vi "ARCOS-- Check  Missing Dependent VI.vi"() -> ()   [LabVIEW 2020]
panel:
  out "DependentVI File":path
  out "ComparedVIs":cluster{string, bool}[](array[cluster])
  out "Missing VIs":string[](array[string])
  out "ExternalAddOn":string[](array[string])
  in  "vi path Compare":path=path "D:/Project/ARCOS2020/ExternalModules/USERCallVISample.vi"
  in  "ARCOSMainVI":path
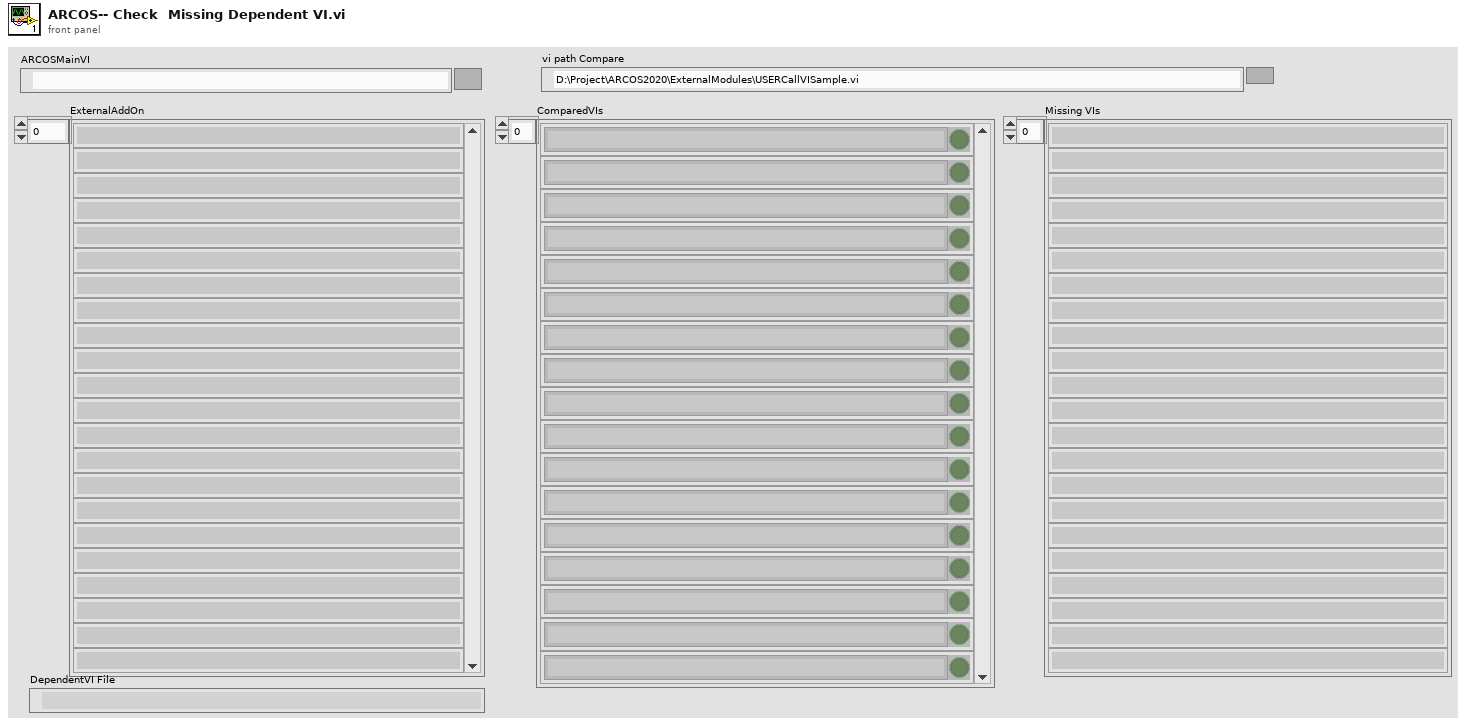
[diagram p1: front panel]
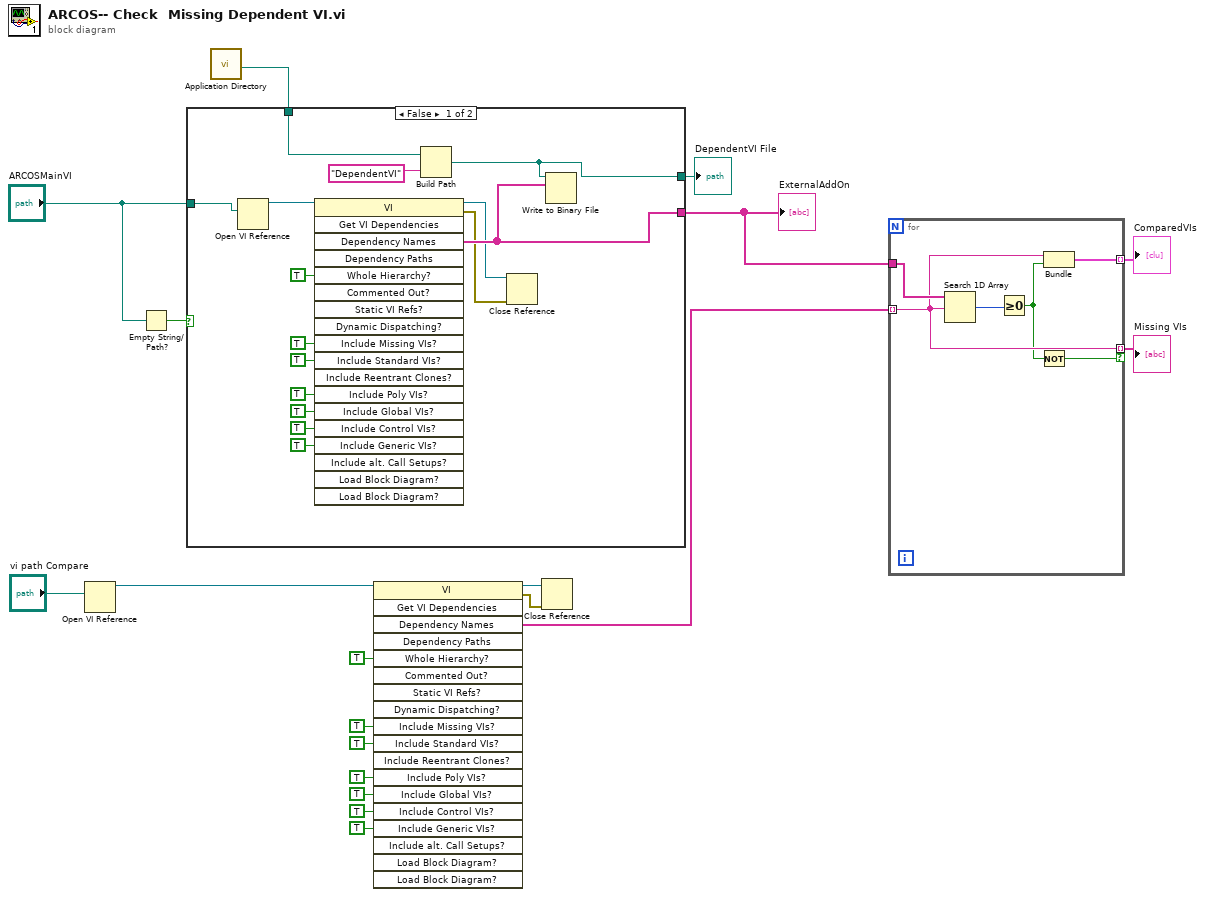
[diagram p0: block diagram]
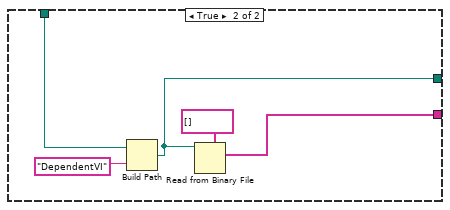
[diagram p2: hidden frame]
diagram:
  n1 = Open VI Reference(vi path="vi path Compare") -> (vi reference=w13:refnum<vi>)  [unwired: 5 in, 1 out]
  n2 = Empty String/Path?(string/path="ARCOSMainVI") -> (empty?=w12:bool)
  n3 = call <vilib>:"Application Directory.vi"() -> ("Application Directory"=w3:path)
  n4 = case shown="False" w12 {
    tunnel: [w26 w37] -> w10
    tunnel: "ARCOSMainVI" -> [w28 _]
    tunnel: w3 -> [w23 w36]
    tunnel: [w22 w35] -> w4
    frame False {
      n5 = Open VI Reference(vi path=w28) -> (vi reference=w29:refnum<vi>)  [unwired: 5 in, 1 out]
      n6 = invoke class="VI" method="Get VI Dependencies"(reference=w29, "Whole Hierarchy?"=TRUE, "Include Missing VIs?"=TRUE ("Include Missing Items?"), "Include Standard VIs?"=TRUE, "Include Poly VIs?"=TRUE, "Include Global VIs?"=TRUE, "Include Control VIs?"=TRUE, "Include Generic VIs?"=TRUE) -> (reference out=w25:refnum<vi>, error out=w24:errorcluster, "Dependency Names"=w26:string[])  [unwired: 11 in, 16 out]
      n7 = Build Path(base path=w23, name or relative path="DependentVI") -> (appended path=w22:path)
      n8 = Close Reference(reference=w25, error in (no error)=w24) -> ()  [unwired: 1 out]
      n9 = Write to Binary File(file (use dialog)=w22, data=w26) -> ()  [unwired: 4 in, 3 out]
    }
    frame True {
      n10 = Build Path(base path=w36, name or relative path="DependentVI") -> (appended path=w35:path)
      n11 = Read from Binary File(5:string[] [] ("Dependency Names"), 11:w35) -> (2:w37:string[])  [unwired: 4 in, 3 out]
    }
  }
  "ExternalAddOn" <- w10
  "DependentVI File" <- w4
  n12 = invoke class="VI" method="Get VI Dependencies"(reference=w13, "Whole Hierarchy?"=TRUE, "Include Missing VIs?"=TRUE ("Include Missing Items?"), "Include Standard VIs?"=TRUE, "Include Poly VIs?"=TRUE, "Include Global VIs?"=TRUE, "Include Control VIs?"=TRUE, "Include Generic VIs?"=TRUE) -> (reference out=w5:refnum<vi>, error out=w6:errorcluster, "Dependency Names"=w11:string[])  [unwired: 11 in, 16 out]
  n13 = Close Reference(reference=w5, error in (no error)=w6) -> ()  [unwired: 1 out]
  n14 = for {
    tunnel: w11 -> [w42] mode=indexing
    tunnel: w10 -> [w44]
    tunnel: [w42] -> w9 mode=indexing if=w43
    tunnel: [w40] -> w7 mode=indexing
    n15 = Search 1D Array(1D array=w44, element=w42) -> (index of element=w45:i32)  [unwired: 1 in]
    n16 = Greater Or Equal To 0?(x=w45) -> (x >= 0?=w41:bool)
    n17 = Not(x=w41) -> (.not. x?=w43:bool)
    n18 = Bundle(w42, w41) -> (w40:cluster{string, bool})  [unwired: 1 in]
  }
  "Missing VIs" <- w9
  "ComparedVIs" <- w7
